vi "Get RegistryKey.vi"(8 "error in (no error)":errorcluster, 11 "SMO":refnum<class "SMO.lvclass">) -> (0 "error out":errorcluster, 2 "RegistryKey":string, 3 "SMO out":refnum<class "SMO.lvclass">)   [LabVIEW 2019, in "SMO.lvclass"]
doc: "JKI State Machine Objects (SMO) 1.3.0.56\nJKI - JKI\nCopyright (c) 2017, JKI"
uses:
  SMO.lvclass
  Support/Attribute.Identity/Attribute.Identity.lvclass
  C:/Users/Patrick/Documents/GitHub/Test (LV2019)/lv-venv/lv.lib/vi.lib/JKI/JKI SMO/Support/Attribute/Attribute.lvclass
  SMO.lvclass/SMO.ctl
  Support/Attribute.Identity/Attribute.Identity.lvclass/Attribute.Identity.ctl
  Support/Attribute/Attribute.lvclass
panel:
  # "For instructions on how to use the JKI State Machine Objects, examples and video tutorials, visit:\nhttp://jki.net/state-machine-objects/\n\nJKI State Machine Objects™\nhttp://jki.net/state-machine-objects/\nCopyright (C) 2005-2015, JKI <info@jki.net>\nALL RIGHTS RESERVED"
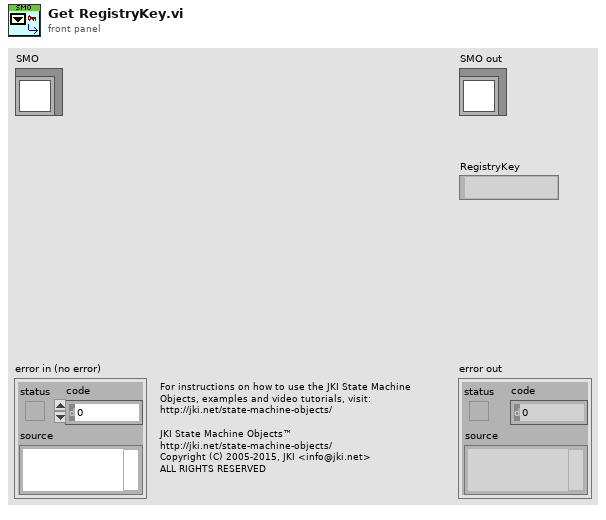
[diagram p1: front panel]
types:
  T1 = typedef "SMO.lvclass/PrivateData--Ref.ctl" = refnum<data-value>
  T2 = typedef "SMO.lvclass/PrivateData--Cluster.ctl" = cluster{"Parent Call":T3, "Registered Processes":T4[], "Sync Notifier":refnum<notifier>, "Process Error Notifier":refnum<notifier>, "Protected Events":T5, "Public Events":T6, "SMO State":T7, "[Dependencies]":T8[], "[Attributes]":refnum<class "Attribute.lvclass">[], "Launcher Close":refnum<notifier>, "Caller Watchdog":refnum<queue>, "Accessibility":T9, "NbStaticDependencies":u32}
  T3 = typedef "SMO.lvclass/Parent Call--Enum.ctl" = enum16{"Allows parent to run", "Does not request parent to run"}
  T4 = typedef "SMO.lvclass/RegisteredProcessData--Cluster.ctl" = cluster{"Name":string, "Static VI Ref":refnum<vi>, "Running":bool, "NotifierRef":u32}
  T5 = typedef "SMO.lvclass/Protected Events.ctl" = cluster{"StopProcesses":refnum<user-event>, "AbortProcesses":refnum<user-event>, "Config Changed":refnum<user-event>, "Dependency":refnum<user-event>}
  T6 = typedef "SMO.lvclass/Public Events.ctl" = cluster{"Error":refnum<user-event>, "State":refnum<user-event>, "Reserve State":refnum<user-event>}
  T7 = typedef "SMO.lvclass/SMOState --Enum.ctl" = enum16{"unknown", "Created", "Started", "Stopped"}
  T8 = typedef "SMO.lvclass/SMO Dependency--Cluster.ctl" = cluster{"Dependency":refnum<class "SMO.lvclass">, "Level":string}
  T9 = typedef "SMO.lvclass/Accessibility--Cluster.ctl" = cluster{"Lock Key":string, "Reserve State":T10}
  T10 = typedef "SMO.lvclass/Reserve State--Enum.ctl" = enum16{"Unreserved", "Reserved", "Self-locked"}
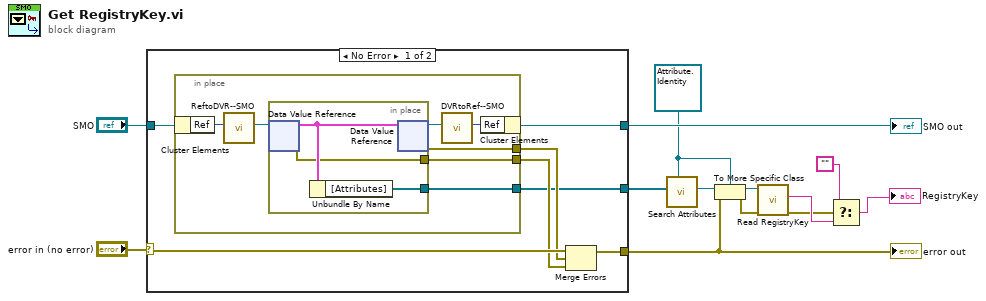
[diagram p0: block diagram]
diagram:
  w8 = refnum<class "Attribute.Identity.lvclass"> refnum ("Attribute.Identity.lvclass")
  n1 = case shown="No Error" "error in (no error)" {
    selector: "error in (no error)" -> [w18 w32]
    tunnel: [w17 w32] -> w7
    tunnel: [w19 w31] -> w11
    tunnel: "SMO" -> [w20 w31]
    tunnel: [w14 _] -> w10
    frame No Error {
      n2 = in-place {
        in-place-border: [w27] -> w14
        in-place-border: [w26] -> w16
        in-place-border: [w25] -> w15
        n3 = in-place-cluster #1(w20) -> ("Ref"=w21:u32)
        n4 = call "ReftoDVR--SMO.vi"("Ref"=w21) -> ("Ref"=w24:T1)  [unwired: 10 in]
        n5 = in-place {
          in-place-border: [w30] -> w27
          in-place-border: [w28] -> w25
          n6 = in-place-dvr #2(w24) -> (w29:T2, w28:errorcluster)
          n7 = Unbundle By Name(w29) -> ("[Attributes]"=w30:refnum<class "Attribute.lvclass">[])
          n8 = in-place-dvr #2(w29) -> (w23:T1, w26:errorcluster)
        }
        n9 = call "DVRtoRef--SMO.vi"("Ref"=w23) -> ("Ref"=w22:u32)  [unwired: 10 in]
        n10 = in-place-cluster #1("Ref"=w22) -> (w19:refnum<class "SMO.lvclass">)
      }
      n11 = Merge Errors(w18, w16, w15) -> (w17:errorcluster)
    }
    frame Error {
    }
  }
  "error out" <- w7
  "SMO out" <- w11
  n12 = call "Search Attributes.vi"("Attribute type"=w8, "[Attributes]"=w10) -> ("Attribute out"=w9:refnum<class "Attribute.lvclass">)  [unwired: 8 in, 1 out]
  n13 = To More Specific Class(target class=w8, reference=w9, error in=w7) -> (specific class reference=w4:refnum<class "Attribute.Identity.lvclass">, error out=w2:errorcluster)
  n14 = call "Read RegistryKey.vi"("error in (no error)"=w2, "Attribute.Identity in"=w4) -> ("error out"=w1:errorcluster, "RegistryKey"=w3:string)  [unwired: 7 in, 1 out]
  n15 = Select(t="", s=w1, f=w3) -> (s? t:f=→"RegistryKey":string)
